vi "Experiment header-Update individual internal element values.vi"(7 "Header file sections":T1=enum."GLOBAL PARAMETERS", 8 "error in (no error)":errorcluster, 9 "Variant":variant, 10 "Name of parameter to update":string, 11 "All header parameters / Header module interface cluster":refnum<vi>) -> (0 "error IO":errorcluster)   [LabVIEW 2017]
uses:
  Typedefs/Header file sections.ctl
  Typedefs/Header parameters cluster-ALL.ctl
  Typedefs/Header subclusters/Header params -Login.ctl
  Typedefs/Header subclusters/Header params-Global Parameters.ctl
  Misc/Experiment Type.ctl
  Typedefs/Header subclusters/Header params-Imaging Modes.ctl
  Typedefs/Header subclusters/Header params-Time Series.ctl
  Typedefs/Header subclusters/Header params-Basic image meta data.ctl
  Typedefs/Frame Size.ctl
  Typedefs/Header subclusters/Header params-Motor Z-stack.ctl
  Typedefs/Header subclusters/Header params-AOL Z-stack.ctl
  Typedefs/Header subclusters/Header params-Functional Imaging.ctl
  Typedefs/Functional Mode.ctl
  Typedefs/AOL modes.ctl
  Typedefs/Plane Mode.ctl
  Typedefs/Header subclusters/Header params-Movement correction.ctl
  Typedefs/Reference source.ctl
  Typedefs/Header subclusters/Header params-Calibration Setup.ctl
  Typedefs/Header subclusters/Header params-statistics.ctl
  Misc/Biology Information.ctl
  Typedefs/Header file type enum.ctl
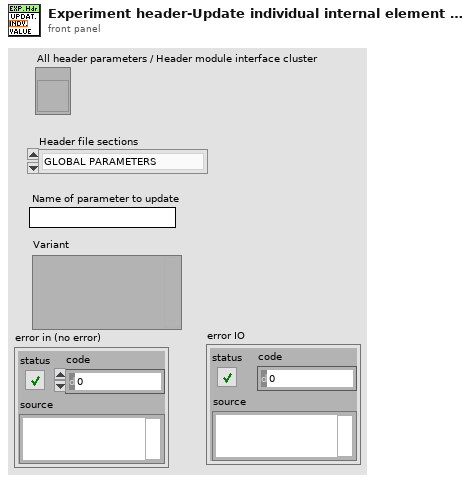
[diagram p1: front panel]
types:
  T1 = typedef "Header file sections.ctl" = enum16{"ALL SECTIONS", "LOGIN", "GLOBAL PARAMETERS", "IMAGING MODES", "TIME SERIES", "MOTOR Z-STACK", "AOL Z-STACK", "FUNCTIONAL IMAGING", "MOVEMENT CORRECTION", "CALIBRATION", "STATISTICS", "BIOLOGY INFORMATION"}
  T2 = typedef "Header file type enum.ctl" = enum16{"All parameters", "Login", "Global Parameters", "Imaging Modes", "Time Series", "Motor Zstack", "AOL Zstack", "Functional Imaging", "Movement Correction", "Calibration Setup", "Statistics", "Biology Information"}
  T3 = typedef "Header file section refs.ctl" = cluster{"Section Name":string, "Section Ref":refnum<vi>, "Section Controls[]":refnum<vi>[]}
  T4 = typedef "Header file parameter names.ctl" = cluster{"Section Name":string, "Array":cluster{"Parameter name":string, "Control ref":refnum<vi>}[]}
  T5 = cluster{"Parameter name":string, "Control ref":refnum<vi>}[]
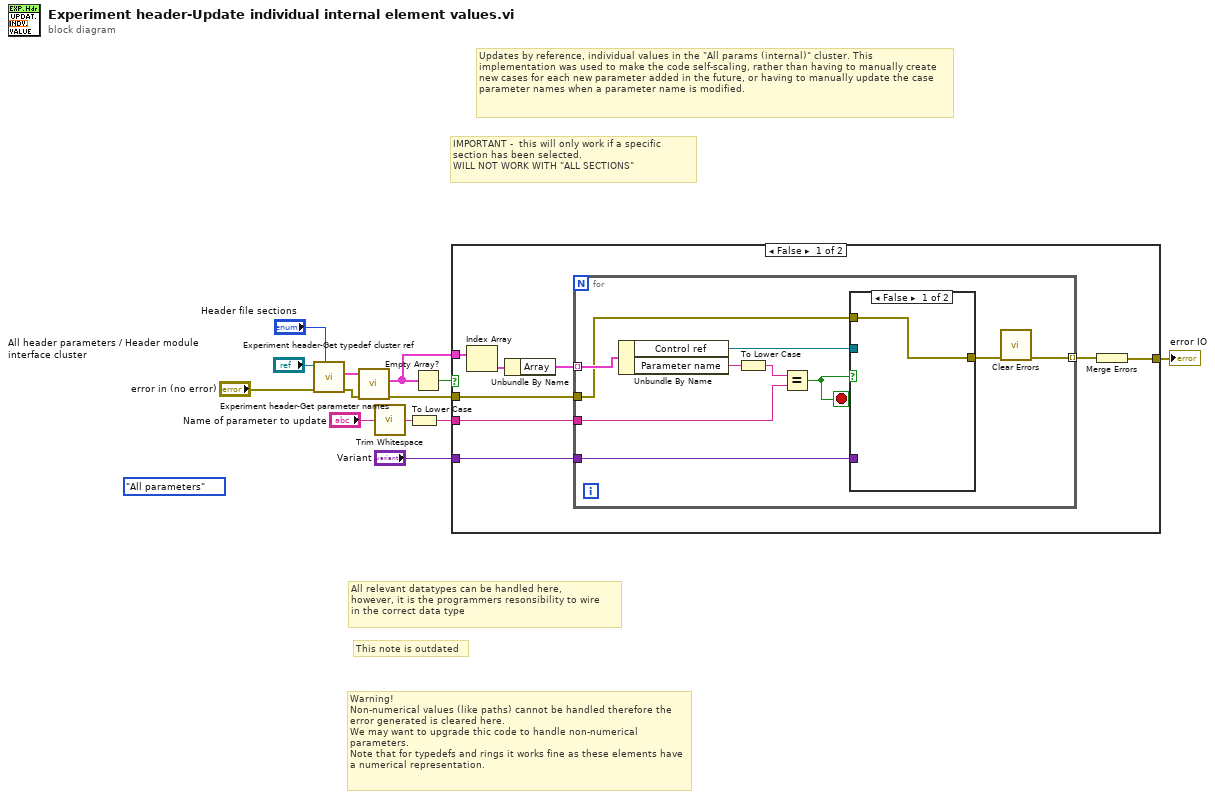
[diagram p0: block diagram]
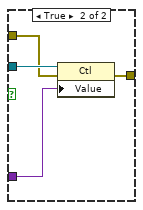
[diagram p2: hidden frame]
diagram:
  (unwired) Header_file_type_enum."All parameters" ("Header file type")
  # "All relevant datatypes can be handled here,\nhowever, it is the programmers resonsibility to wire\nin the correct data type"
  # "This note is outdated"
  # "IMPORTANT -  this will only work if a specific \nsection has been selected. \nWILL NOT WORK WITH \"ALL SECTIONS\""
  # "Warning!\nNon-numerical values (like paths) cannot be handled therefore the error generated is cleared here.\nWe may want to upgrade thic code to handle non-numerical parameters.\nNote that for typedefs and rings it works fine as these elements have a numerical representation."
  # "Updates by reference, individual values in the \"All params (internal)\" cluster. This implementation was used to make the code self-scaling, rather than having to manually create new cases for each new parameter added in the future, or having to manually update the case parameter names when a parameter name is modified."
  n1 = call "Experiment header-Get typedef cluster ref.vi"("Header file sections"="Header file sections", "error in (no error)"="error in (no error)", "All header parameters / Header module interface cluster"="All header parameters / Header module interface cluster") -> ("error out"=w2:errorcluster, "Section Refs"=w10:T3[])  [unwired: 5 in, 2 out]
  n2 = call "Experiment header-Get parameter names.vi"("error in (no error)"=w2, "Section Refs"=w10) -> ("error out"=w1:errorcluster, "All Parameter names"=w7:T4[])  [unwired: 7 in, 1 out]
  n3 = call <vilib>:"Trim Whitespace.vi"("string"="Name of parameter to update") -> ("trimmed string"=w12:string)  [unwired: 1 in]
  n4 = To Lower Case(string=w12) -> (all lower case string=w6:string)
  n5 = Empty Array?(array=w7) -> (empty?=w8:bool)
  n6 = case shown="False" w8 {
    tunnel: w7 -> [w21 _]
    tunnel: w6 -> [w18 _]
    tunnel: "Variant" -> [w17 _]
    tunnel: [w15 w37] -> w4
    tunnel: w1 -> [w14 w37]
    frame False {
      n7 = Index Array(array=w21) -> (element=w20:T4)  [unwired: 1 in]
      n8 = Unbundle By Name(w20) -> ("Array"=w19:T5)
      n9 = for {
        tunnel: w19 -> [w31] mode=indexing
        tunnel: w18 -> [w28]
        tunnel: w17 -> [w25]
        tunnel: [w23] -> w16 mode=indexing
        tunnel: w14 -> [w22]
        stop <- w27 stop-if-true
        n10 = Unbundle By Name(w31) -> ("Control ref"=w26:refnum<vi>, "Parameter name"=w30:string)
        n11 = To Lower Case(string=w30) -> (all lower case string=w29:string)
        n12 = Equal?(x=w29, y=w28) -> (x = y?=w27:bool)
        n13 = case shown="False" w27 {
          tunnel: w26 -> [_ w36]
          tunnel: w25 -> [_ w35]
          tunnel: [w32 w34] -> w24
          tunnel: w22 -> [w32 w33]
          frame False {
          }
          frame True {
            n14 = property class="Ctl"(reference=w36, error in=w33, "Value"=w35) -> (error out=w34:errorcluster)  [unwired: 1 out]
          }
        }
        n15 = call <vilib>:"Clear Errors.vi"("error in (no error)"=w24) -> ("error out"=w23:errorcluster)  [unwired: 5 in, 1 out]
      }
      n16 = Merge Errors(w16) -> (w15:errorcluster)
    }
    frame True {
    }
  }
  "error IO" <- w4
